vi "angleSetpointFix.vi"(7 "maxDiff":dbl=0.5, 11 "Angle in":dbl) -> (3 "Angle out":dbl)   [LabVIEW 2016]
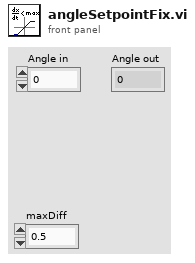
[diagram p1: front panel]
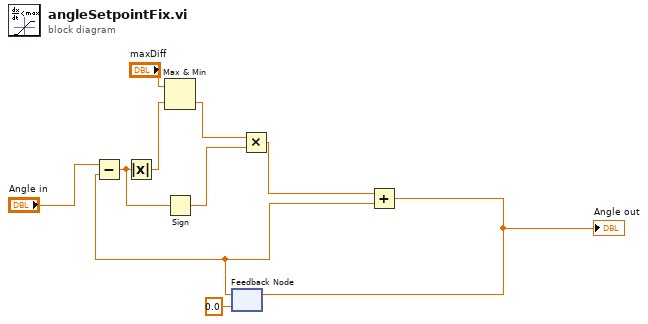
[diagram p0: block diagram]
diagram:
  n1 = feedback #1(0.0) -> (w3:dbl)
  n2 = Subtract(x="Angle in", y=w3) -> (x-y=w7:dbl)
  n3 = Absolute Value(x=w7) -> (abs(x)=w10:dbl)
  n4 = Max & Min(x="maxDiff", y=w10) -> (min(x,y)=w6:dbl)  [unwired: 1 out]
  n5 = Sign(1:w7) -> (0:w5:dbl)
  n6 = Multiply(x=w6, y=w5) -> (x*y=w4:dbl)
  n7 = Add(x=w4, y=w3) -> (x+y=w2:dbl)
  "Angle out" <- w2
  n8 = feedback-in #1(w2) -> ()
